vi "Configure Output Inhibit Mode.vi"(8 "error in (no error)":errorcluster, 10 "Mode(0:Latching)":u16(ring) items=["Latching", "Live", "OFF"], 11 "VISA resource name":refnum<visa-resource-name>) -> (0 "error out":errorcluster, 3 "VISA resource name out":refnum<visa-resource-name>)   [LabVIEW 2015, in "IT6000C.lvlib"]
doc: "This command sets the forbidden output mode for digital IO.The corresponding functions of different options are detailed in the description of IO -- 5. Inh-living, not-invert in the user's manual.\n\n0:Latching\n1:LIVE\n2:OFF"
uses:
  <instrlib>/IT6000C/IT6000C.lvlib
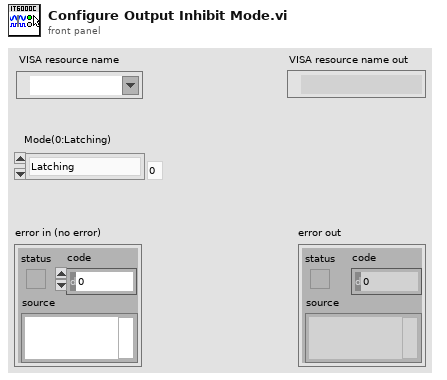
[diagram p1: front panel]
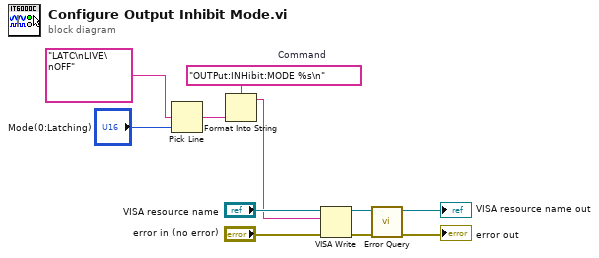
[diagram p0: block diagram]
diagram:
  w5 = "OUTPut:INHibit:MODE %s\n"  # Command
  n1 = Pick Line(multi-line string="LATC\nLIVE\nOFF", line index="Mode(0:Latching)") -> (output string=w1:string)  [unwired: 1 in]
  n2 = Format Into String(format string=w5, w1) -> (resulting string=w4:string)  [unwired: 2 in, 1 out]
  n3 = VISA Write(VISA resource name="VISA resource name", write buffer=w4, error in (no error)="error in (no error)") -> (VISA resource name out=w8:refnum<visa-resource-name>, error out=w9:errorcluster)  [unwired: 1 out]
  n4 = call <instrlib>:"Error Query.vi"("error in (no error)"=w9, "VISA resource name"=w8) -> ("error out"=→"error out":errorcluster, "VISA resource name out"=→"VISA resource name out":refnum<visa-resource-name>)  [unwired: 6 in, 2 out]
